vi "Login Main.vi"() -> (2 "User":string)   [LabVIEW 2022 SP3]
uses:
  <vilib>/Utility/file.llb/Read Delimited Spreadsheet (string).vi
panel:
  out "Role":string
  out "error out":errorcluster
  in  "error in":errorcluster
  out "Verify Auth":bool
  out "Tab Control":enum32{"Page 1", "Page 2"}(tab)
  in  "EXIT":bool
  in  "Log-In":bool
  in  "USER NAME":string(combo)
  in  "PASSWORD":string
  in  "Show Password":bool
  in  "Change Password":bool
  in  "Change":bool
  in  "NEW PASSWORD":string
  in  "OLD PASSWORD":string
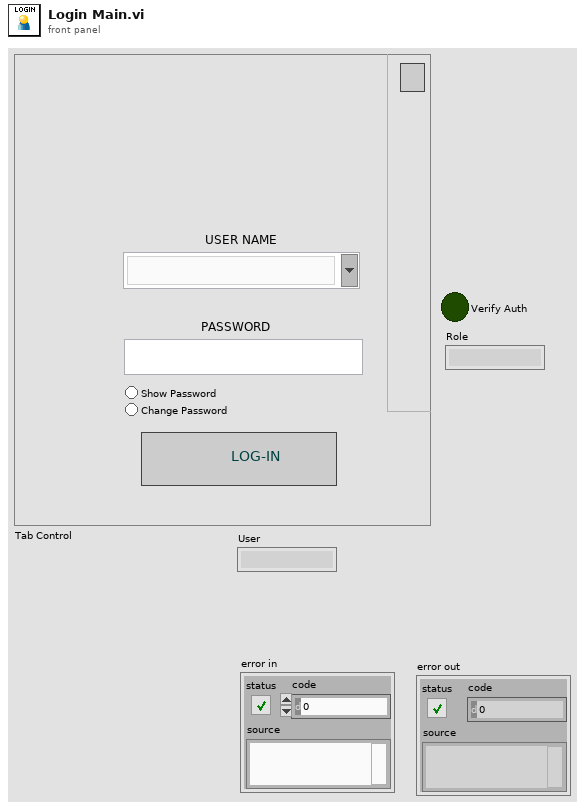
[diagram p1: front panel]
types:
  T1 = enum16{"Initialize", "Poll", "Login", "Move 2 Page", "Change Password", "Wrong Password", "Exit"}
  T2 = cluster{"User Name":string, "Password":string, "ROLE":string}
  T3 = typedef "SeCrTs-file folder ctl.ctl" = cluster{"Datalog path":path, "Configuration path":path, "Signal list path":path, "Sub vi's":path, "Authentication":path, "Sequence":path, "Event Log":path, "CS Error log":path, "RT Error Log":path}
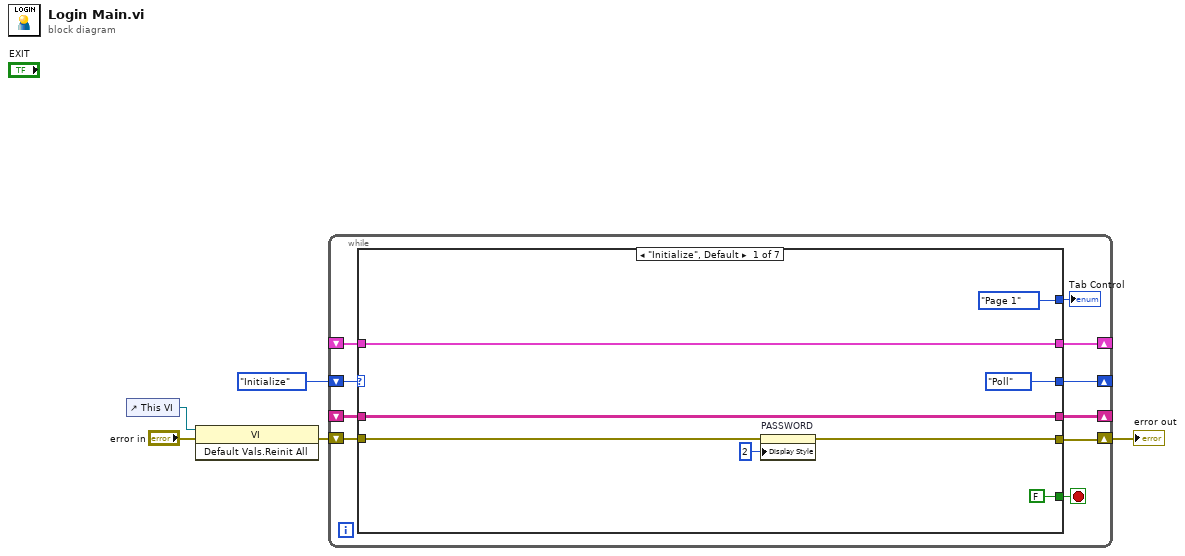
[diagram p0: block diagram]
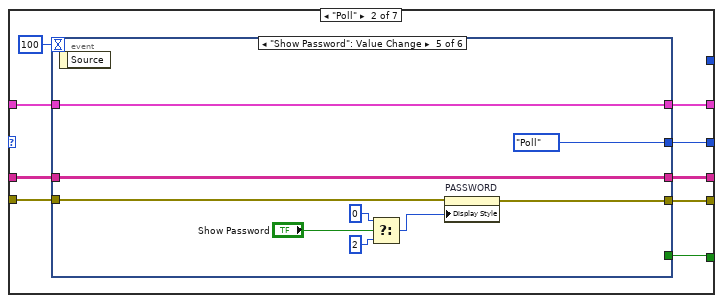
[diagram p2: hidden frame]
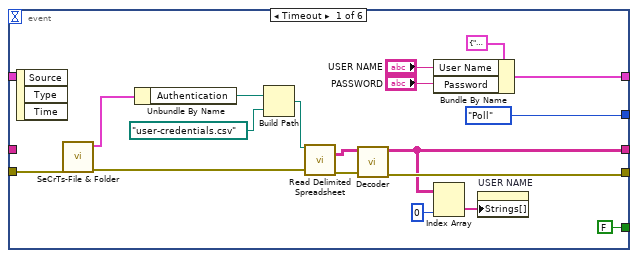
[diagram p3: hidden frame]
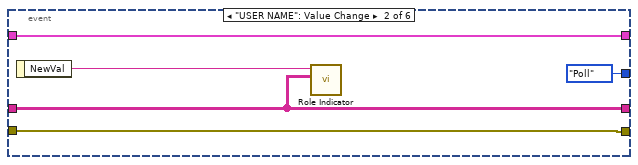
[diagram p4: hidden frame]
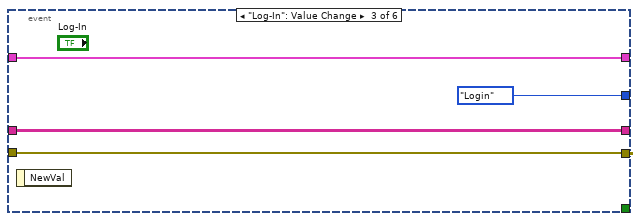
[diagram p5: hidden frame]
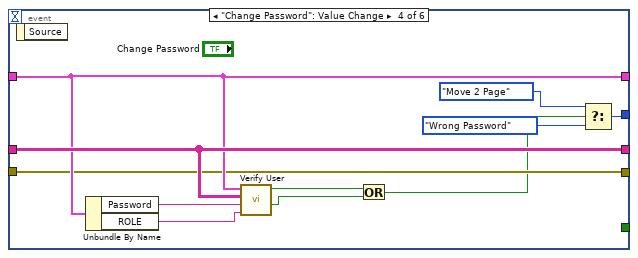
[diagram p6: hidden frame]
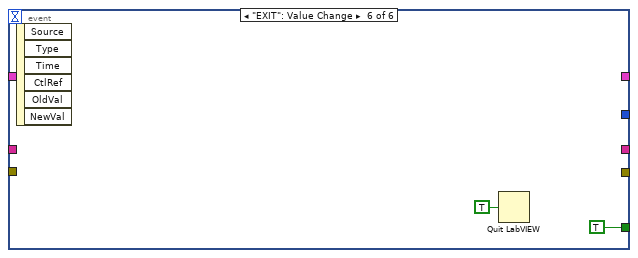
[diagram p7: hidden frame]
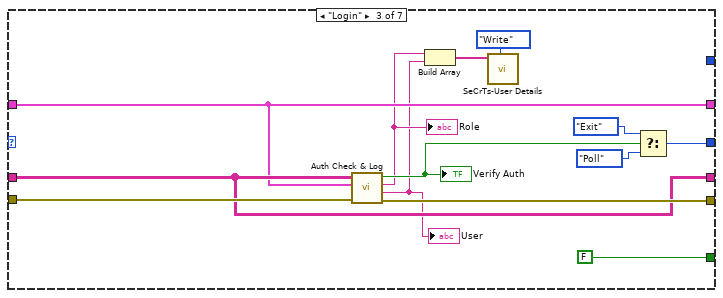
[diagram p8: hidden frame]
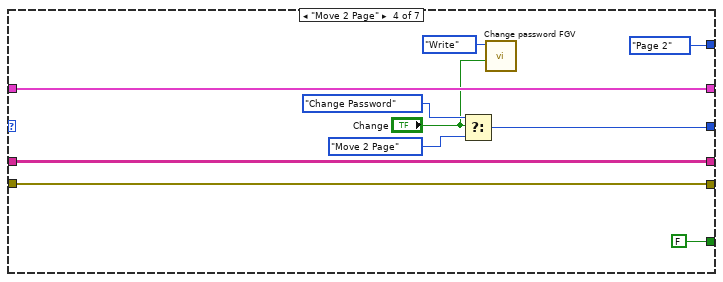
[diagram p9: hidden frame]
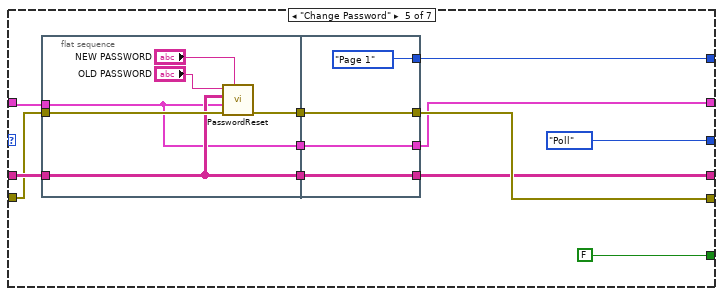
[diagram p10: hidden frame]
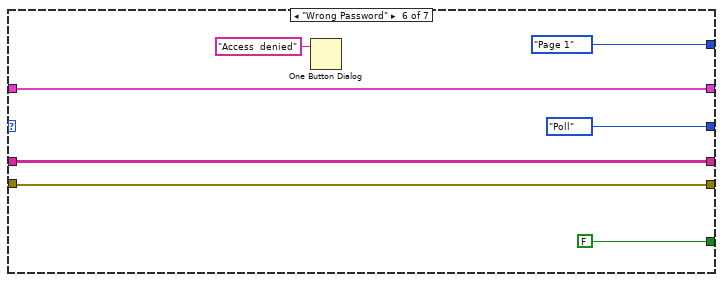
[diagram p11: hidden frame]
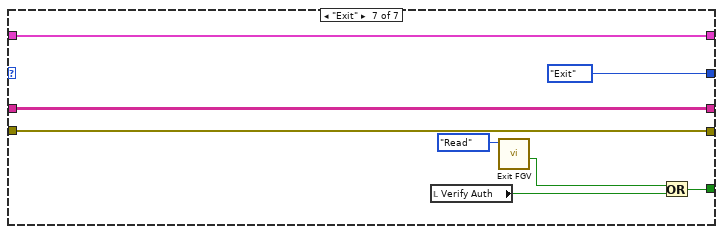
[diagram p12: hidden frame]
diagram:
  n1 = control-ref of="This VI"() -> (w5:refnum<vi>)
  n2 = invoke class="VI" method="Default Vals.Reinit All"(reference=w5, error in="error in") -> (error out=w3:errorcluster)  [unwired: 1 in, 2 out]
  n3 = while {
    shift-right: [w11] -> w1
    shift-left: w3 -> [w12]
    shift-right: [w13] -> _
    shift-left: T1."Initialize" -> [w15]
    shift-right: [w10] -> _
    shift-left: _ -> [w8]
    shift-right: [w9] -> _
    shift-left: _ -> [w7]
    stop <- w6 stop-if-true
    n4 = case shown="\"Initialize\", Default" w15 {
      tunnel: [enum32{"Page 1", "Page 2"}."Page 1" ("Tab Control") _ _ enum32{"Page 1", "Page 2"}."Page 2" ("Tab Control") w113 enum32{"Page 1", "Page 2"}."Page 1" ("Tab Control") _] -> w14
      tunnel: [T1."Poll" w28 w89 w99 T1."Poll" ("f") T1."Poll" ("f") T1."Exit" ("f")] -> w13
      tunnel: w12 -> [w18 w32 w93 w101 w114 w128 w138]
      tunnel: [w17 w31 w94 w101 w111 w128 w138] -> w11
      tunnel: [w21 w29 w91 w103 w106 w131 w141] -> w10
      tunnel: [w20 w27 w92 w102 w108 w130 w139] -> w9
      tunnel: w8 -> [w21 w26 w91 w103 w115 w131 w141]
      tunnel: w7 -> [w20 w25 w92 w102 w116 w130 w139]
      tunnel: [FALSE w24 FALSE FALSE FALSE FALSE w137] -> w6
      frame "Initialize", Default {
        n5 = property on="PASSWORD" class="Str"(error in=w18, "Display Style"=u32 2) -> (error out=w17:errorcluster)  [unwired: 1 in, 1 out]
      }
      frame "Poll" {
        n6 = event shown="[4] \"Show Password\": Value Change" {
          selector: _ -> [_ _ _ _ _ _]
          dyn-events: _ -> [_ _ _ _ _ _]
          timeout: 100 -> [_ _ _ _ _ _]
          tunnel: w32 -> [w36 w54 w56 w67 w76 _]
          tunnel: [w45 w54 w56 w67 w77 _] -> w31
          tunnel: [w42 w55 w58 w69 w79 _] -> w29
          tunnel: [T1."Poll" T1."Poll" ("f") T1."Login" w66 T1."Poll" ("f") _] -> w28
          tunnel: [w40 w52 w57 w70 w78 _] -> w27
          tunnel: w26 -> [_ w55 w58 w69 w79 _]
          tunnel: w25 -> [_ w52 w57 w70 w78 _]
          tunnel: [FALSE _ _ _ _ TRUE] -> w24
          event Timeout {
            n7 = event-data() -> ()  [unwired: 1 in, 3 out]
            n8 = call "SeCrTs-File & Folder.vi"("error in (no error)"=w36) -> ("error out"=w35:errorcluster, "File Output"=w34:T3)  [unwired: 9 in]
            n9 = Unbundle By Name(w34) -> ("Authentication"=w50:path)
            n10 = Build Path(base path=w50, name or relative path=path "user-credentials.csv") -> (appended path=w48:path)
            n11 = call-poly <vilib>:"Read Delimited Spreadsheet.vi"("file path (dialog if empty)"=w48, "error in (no error)"=w35) -> ("all rows"=w47:string[][], "error out"=w46:errorcluster)  [unwired: 8 in, 4 out]
            n12 = call "Decoder.vi"("error in"=w46, "Encoded Data"=w47) -> ("error out"=w45:errorcluster, "Decoded Data"=w40:string[][])  [unwired: 8 in]
            n13 = Bundle By Name(cluster=T2 {"User Name"="", "Password"="", "ROLE"=""}, "User Name"="USER NAME", "Password"="PASSWORD") -> (w42:T2)
            n14 = Index Array(array=w40, index (col)=0 ("index (row)")) -> (element=w38:string[])  [unwired: 1 in]
            n15 = property on="USER NAME" class="CmbBox"("Strings[]"=w38) -> ()  [unwired: 2 in, 2 out]
          }
          event "USER NAME": Value Change {
            n16 = event-data() -> ("NewVal"=w53:string)  [unwired: 1 in]
            n17 = call "Role Indicator.vi"("Decoded Data"=w52, "NewVal"=w53) -> ()  [unwired: 9 in, 1 out]
          }
          event "Log-In": Value Change {
            n18 = event-data() -> ()  [unwired: 1 in, 1 out]
          }
          event "Change Password": Value Change {
            n19 = event-data() -> ()  [unwired: 1 in, 1 out]
            n20 = Unbundle By Name(w69) -> ("Password"=w68:string, "ROLE"=w60:string)
            n21 = call "Verify User.vi"("ROLE"=w60, "OLD PASSWORD in"=w68, "Authenticated Data"=w70, "User Cred"=w69) -> ("Administator?"=w62:bool, "Password True?"=w63:bool)  [unwired: 5 in, 1 out]
            n22 = Or(x=w63, y=w62) -> (x .or. y?=w61:bool)
            n23 = Select(t=T1."Move 2 Page", s=w61, f=T1."Wrong Password") -> (s? t:f=w66:T1)
          }
          event "Show Password": Value Change {
            n24 = event-data() -> ()  [unwired: 1 in, 1 out]
            n25 = Select(t=0, s="Show Password", f=2) -> (s? t:f=w72:i32)
            n26 = property on="PASSWORD" class="Str"(error in=w76, "Display Style"=w72) -> (error out=w77:errorcluster)  [unwired: 1 in, 1 out]
          }
          event "EXIT": Value Change {
            n27 = event-data() -> ()  [unwired: 1 in, 6 out]
            n28 = Quit LabVIEW(quit? (T)=TRUE) -> ()
          }
        }
      }
      frame "Login" {
        n29 = call "Auth Check & Log.vi"("error in"=w93, "User Cred"=w91, "Authenticated Data"=w92) -> ("error out"=w94:errorcluster, "User"=w83:string, "Role Out"=w84:string, "Verify Auth"=w86:bool)  [unwired: 5 in]
        "Verify Auth" <- w86
        "Role" <- w84
        "User" <- w83
        n30 = Build Array(w84, w83) -> (w82:string[])
        n31 = call "SeCrTs-User Details.vi"("Enum"=enum16{"Read", "Write"}."Write", "User details"=w82) -> ()  [unwired: 8 in, 2 out]
        n32 = Select(t=T1."Exit", s=w86, f=T1."Poll") -> (s? t:f=w89:T1)
      }
      frame "Move 2 Page" {
        n33 = Select(t=T1."Change Password", s="Change", f=T1."Move 2 Page") -> (s? t:f=w99:T1)
        n34 = call "Change password FGV.vi"("Change Password in"="Change", "Enum"=enum16{"Read", "Write"}."Write") -> ()  [unwired: 8 in, 2 out]
      }
      frame "Change Password" {
        n35 = flat-sequence {
          tunnel: w116 -> [w118]
          tunnel: w115 -> [w117]
          tunnel: w114 -> [w120]
          tunnel: [w119] -> w112
          tunnel: [w118] -> w109
          tunnel: [w117] -> w107
          tunnel: [enum32{"Page 1", "Page 2"}."Page 1" ("Tab Control")] -> w113
          tunnel: w112 -> [w125]
          tunnel: [w125] -> w111
          tunnel: w109 -> [w124]
          tunnel: [w124] -> w108
          tunnel: [w123] -> w106
          tunnel: w107 -> [w123]
          frame #0 {
            n36 = call "PasswordReset.vi"("NEW PASSWORD"="NEW PASSWORD", "error in"=w120, "User Cred"=w117, "Authenticated Data"=w118, "OLD PASSWORD"="OLD PASSWORD") -> ("error out"=w119:errorcluster)  [unwired: 6 in]
          }
          frame #1 {
          }
        }
      }
      frame "Wrong Password" {
        n37 = One Button Dialog(message="Access  denied") -> ()  [unwired: 1 in, 1 out]
      }
      frame "Exit" {
        n38 = local read "Verify Auth"() -> (w134:bool)
        n39 = call "Exit FGV.vi"("Enum"=enum16{"Read", "Write"}."Read") -> ("Exit Out"=w135:bool)  [unwired: 10 in]
        n40 = Or(x=w135, y=w134) -> (x .or. y?=w137:bool)
      }
    }
    "Tab Control" <- w14
  }
  "error out" <- w1
